vi "Extract the Sine Wave NEW FILTER.vi"() -> ()   [LabVIEW 2019, in "DSP.lvclass"]
doc: "This example demonstrates how a signal can be extracted from bandlimited noise using the filter VIs."
uses:
  DSP.lvclass
  <vilib>/Analysis/3filter.llb/Filter Passband Type.ctl
  <vilib>/Analysis/3filter.llb/IIR Cascade Filter with I.C. (DBL).vi
  <vilib>/Analysis/3filter.llb/IIR Filter with I.C. (DBL).vi
  <vilib>/addons/Digital Filter Design/Process.llb/DFD Filtering with State (Wfm).vi
  <vilib>/addons/Digital Filter Design/Process.llb/DFD Filtering (Wfm NChan).vi
  <vilib>/Analysis/3filter.llb/Butterworth Filter (DBL).vi
  <vilib>/Analysis/NI_AALBase.lvlib
  <vilib>/addons/Digital Filter Design/NI_DigFilterLicensed.lvlib
  <vilib>/measure/NI_MABase.lvlib
panel:
  in  "Q":dbl
  in  "notch (Hz)":dbl
  out "Numeric":i32
  out "Waveform Graph":cluster{dbl, dbl, "Filtered X":dbl[]}[](graph)
  in  "Sample rate (Hz)":dbl=1000.0
  in  "Stop":bool
  in  "Filter Order":i32(slide)=5 scale=0.0..10.0
  in  "Cut-Off Frequency (Hz)":dbl(slide)=20.0 scale=0.0..100.0
  in  "Sine Frequency (Hz)":dbl(slide)=10.0 scale=0.0..200.0
  # "Overview: Removes additive noise from a sinusoid using a lowpass filter.\nRequirements: LabVIEW Full Development System\nInstructions:\n1. Run the VI.\n2. Change the Cut-Off Frequency and Filter Order, noting the effect on the filtered waveform.\n3. Click Stop to stop the VI."
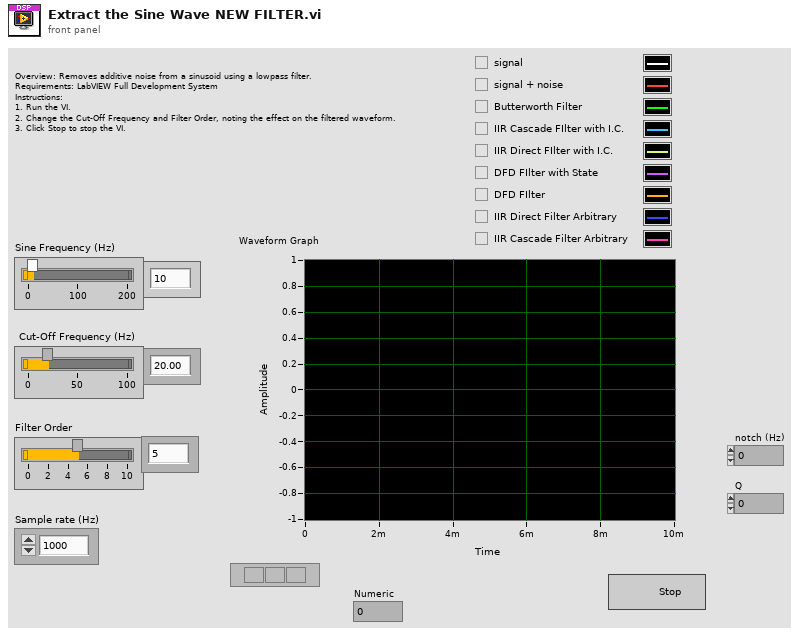
[diagram p1: front panel]
types:
  T1 = cluster{"filter structure":enum32{"IIR 2nd Order", "IIR 4th Order"}, "Reverse Coefficients":dbl[], "Forward Coefficients":dbl[]}
  T2 = enum16{"Sine Wave", "Triangle Wave", "Square Wave", "Sawtooth Wave"}
  T3 = typedef "NI_AALBase.lvlib/Filter Passband Type.ctl" = enum32{"Lowpass", "Highpass", "Bandpass", "Bandstop"}
  T4 = typedef "NI_DigFilterLicensed.lvlib/DFD Filter Obj.ctl" = cluster{"mSRate_Fs":dbl, "mSRate_Version":string, "mSRate_Comments":string, "mSRate_OrgCoef":T5, "mSRate_CurCoef":T5, "mSRate_Quantized?":bool, "mSRate_QCoef":T5, "mSRate_QSettings":T7[], "mSRate_Order":i32, "mSRate_Scaling":cluster{"mSRate_ScaleByPowerOf2?":bool, "mSRate_ScaleType":T9}}
  T5 = typedef "NI_DigFilterLicensed.lvlib/DFD Filter Coef.ctl" = cluster{"type":T6, "gain":dbl, "coef a (k)":dbl[], "coef b (v)":dbl[]}
  T6 = typedef "NI_DigFilterLicensed.lvlib/DFD Filter Structure Type Selector.ctl" = enum16{"Undefined", "FIR Direct Form", "FIR Direct Form Transposed", "FIR Symmetric", "FIR Antisymmetric", "IIR Direct Form I", "IIR Direct Form I Transposed", "IIR Direct Form II", "IIR Direct Form II Transposed", "IIR Cascaded Second Order Sections Form I", "IIR Cascaded Second Order Sections Form I Transposed", "IIR Cascaded Second Order Sections Form II", "IIR Cascaded Second Order Sections Form II Transposed", "Lattice Allpass (basic sections)", "Lattice Allpass (one multiplier sections)", "Lattice Allpass (normalized sections)", "Lattice AR (basic sections)", "Lattice AR (one multiplier sections)", "Lattice AR (normalized sections)", "Lattice MA (minimum phase)", "Lattice MA (maximum phase)", "Lattice ARMA (basic sections)", "Lattice ARMA (one multiplier sections)", "Lattice ARMA (normalized sections)"}
  T7 = typedef "NI_DigFilterLicensed.lvlib/dfd_Internal Quantization Settings.ctl" = cluster{"source":T8, "wl":i16, "iwl":i16, "overflow mode":enum16{"Saturation", "Wrap"}, "rounding mode":enum16{"Nearest", "Truncation"}, "signed?":bool}
  T8 = typedef "NI_DigFilterLicensed.lvlib/dfd_Internal Quantization Srcs.ctl" = u16
  T9 = typedef "NI_DigFilterLicensed.lvlib/DFD Coef Norm Type.ctl" = enum16{"No Norm", "Time Domain 1-Norm", "Time Domain 2-Norm", "Time Domain Inf-Norm"}
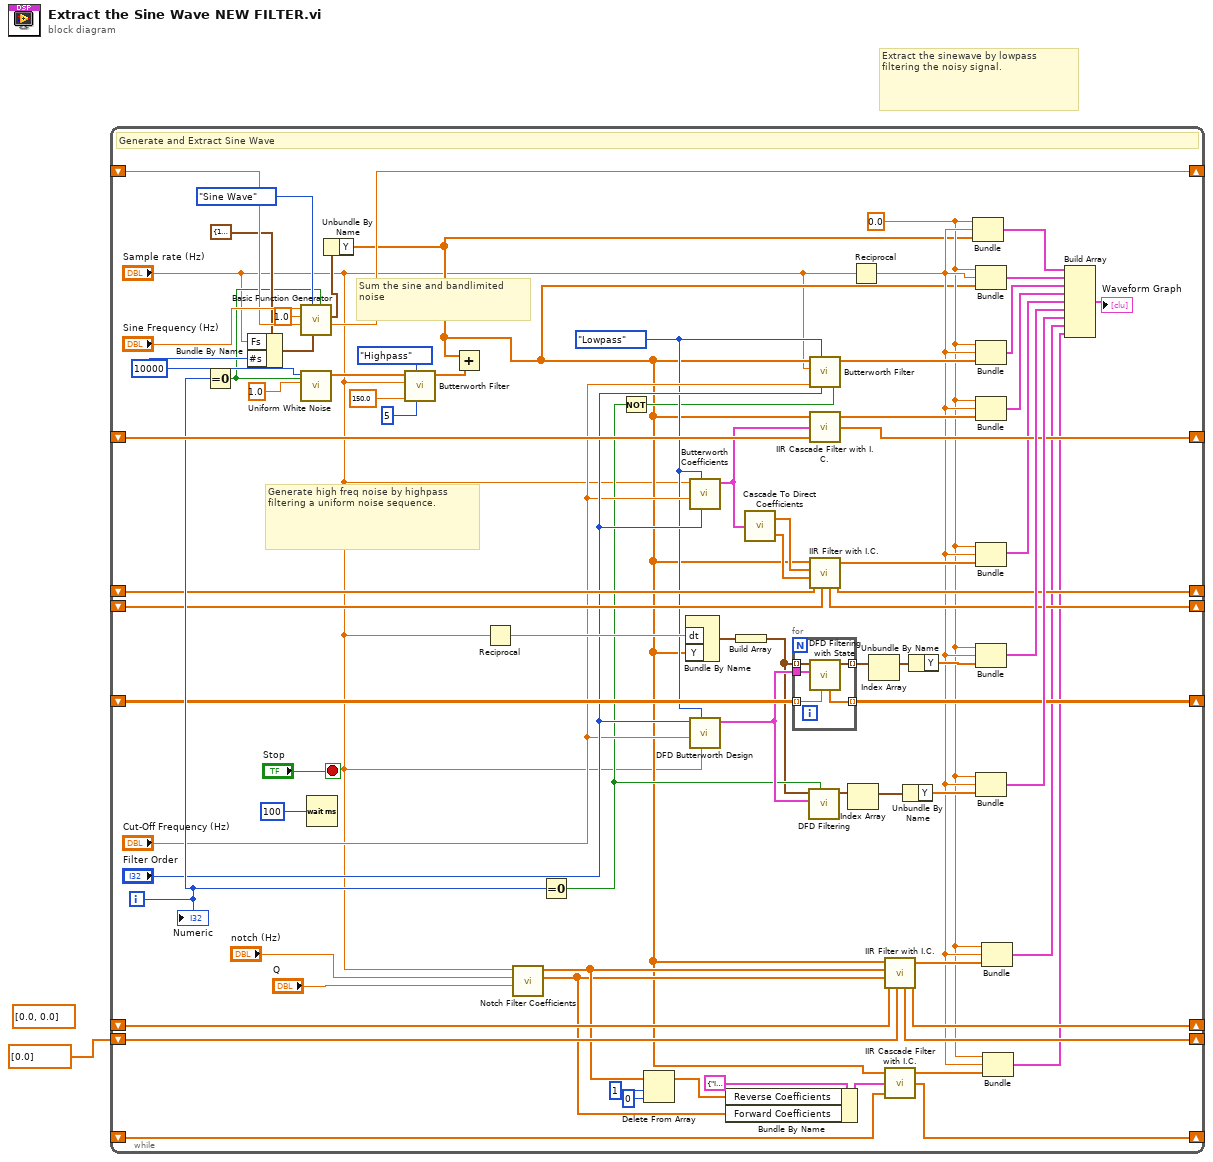
[diagram p0: block diagram]
diagram:
  (unwired) dbl[] [0.0, 0.0] ("Final X Conditions")
  # "Extract the sinewave by lowpass filtering the noisy signal."
  n1 = while {
    shift-right: [w62] -> _
    shift-left: _ -> [w72]
    shift-right: [w64] -> _
    shift-left: _ -> [w63]
    shift-right: [w57] -> _
    shift-left: _ -> [w55]
    shift-right: [w56] -> _
    shift-left: _ -> [w54]
    shift-right: [w23] -> _
    shift-left: _ -> [w35]
    shift-right: [w36] -> _
    shift-left: dbl[] [0.0] ("Final X Conditions") -> [w34]
    shift-right: [w32] -> _
    shift-left: _ -> [w31]
    shift-right: [w5] -> _
    shift-left: _ -> [w17]
    i -> [w71]
    stop <- "Stop" stop-if-true
    w13 = 0.0
    w41 = Filter_Passband_Type."Lowpass" ("filter type")
    w28 = 10000
    # "Sum the sine and bandlimited noise"
    # "Generate high freq noise by highpass filtering a uniform noise sequence."
    # "Generate and Extract Sine Wave"
    n2 = Equal To 0?(x=w71) -> (x = 0?=w24:bool)
    n3 = Bundle By Name(cluster=cluster{"Fs":dbl, "#s":dbl} {"Fs"=1000.0, "#s"=1000.0} ("sampling info"), "Fs"="Sample rate (Hz)", "#s"=w28) -> (w27:cluster{"Fs":dbl, "#s":dbl})
    n4 = call <vilib>:"Basic Function Generator.vi"("reset signal"=w24, "sampling info"=w27, "signal type"=T2."Sine Wave", "phase"=w31, "amplitude"=1.0, "frequency"="Sine Frequency (Hz)") -> ("phase out"=w32:dbl, "signal out"=w25:waveform(dbl))  [unwired: 3 in, 1 out]
    n5 = call <vilib>:"Uniform White Noise.vi"("initialize?"=w24, "amplitude"=1.0, "samples"=w28) -> ("uniform white noise"=w50:dbl[])  [unwired: 7 in, 1 out]
    n6 = Wait (ms)(milliseconds to wait=u32 100) -> ()  [unwired: 1 out]
    n7 = Unbundle By Name(w25) -> ("Y"=w4:dbl[])
    n8 = call-poly <vilib>:"Butterworth Filter.vi"("order"=5, "filter type"=Filter_Passband_Type."Highpass", "low cutoff freq: fl"=150.0, "sampling freq: fs"="Sample rate (Hz)", "X"=w50) -> ("Filtered X"=w49:dbl[])  [unwired: 3 in, 1 out]
    n9 = Add(x=w4, y=w49) -> ()  [unwired: 1 out]
    n10 = Reciprocal(x="Sample rate (Hz)") -> (1/x=w53:dbl)
    n11 = call "Notch Filter Coefficients.vi"("Q"="Q", "notch (Hz)"="notch (Hz)", "Sample rate (Hz)"="Sample rate (Hz)") -> ("Forward Coefficients"=w8:dbl[], "Reverse Coefficients"=w9:dbl[])  [unwired: 7 in]
    n12 = Equal To 0?(x=w71) -> (x = 0?=w39:bool)
    n13 = Not(x=w39) -> (.not. x?=w40:bool)
    n14 = Delete From Array(array=w9, length=1, index=0) -> (array with subset deleted=w12:dbl[])  [unwired: 1 out]
    n15 = Bundle By Name("dt"=w53, "Y"=w4) -> (w7:waveform(dbl))  [unwired: 1 in]
    n16 = call <vilib>:"Butterworth Coefficients.vi"("order"="Filter Order", "filter type"=w41, "low cutoff freq: fl"="Cut-Off Frequency (Hz)", "sampling freq: fs"="Sample rate (Hz)") -> ("IIR Filter Cluster"=w22:T1)  [unwired: 6 in, 1 out]
    n17 = call <vilib>:"DFD Butterworth Design.vi"("fs [Hz]"="Sample rate (Hz)", "filter type"=w41, "low cutoff freq [Hz]"="Cut-Off Frequency (Hz)", "order"="Filter Order") -> ("filter out"=w52:T4)  [unwired: 6 in, 1 out]
    n18 = Bundle By Name(cluster=T1 {"filter structure"=enum."IIR 2nd Order", "Reverse Coefficients"=[], "Forward Coefficients"=[]} ("IIR Filter Cluster"), "Reverse Coefficients"=w12, "Forward Coefficients"=w8) -> (w21:T1)
    n19 = Build Array(w7) -> (w6:waveform(dbl)[])
    n20 = call <vilib>:"Cascade To Direct Coefficients.vi"("IIR Filter Cluster"=w22) -> ("Reverse Coefficients"=w59:dbl[], "Forward Coefficients"=w58:dbl[])
    n21 = for {
      tunnel: [w85] -> w64 mode=indexing
      tunnel: w63 -> [w84] mode=indexing
      tunnel: w52 -> [w83]
      tunnel: w6 -> [w82] mode=indexing
      tunnel: [w81] -> w44 mode=indexing
      n22 = call-poly <vilib>:"DFD Filtering with State.vi"("state in"=w84, "filter"=w83, "signal in"=w82) -> ("signal out"=w81:waveform(dbl), "state out"=w85:dbl[])  [unwired: 6 in, 1 out]
    }
    n23 = call-poly <vilib>:"DFD Filtering.vi"("init? (F)"=w39, "filter"=w52, "signal in"=w6) -> ("signal out"=w46:waveform(dbl)[])  [unwired: 7 in, 1 out]
    n24 = call-poly <vilib>:"Butterworth Filter.vi"("init/cont (init:F)"=w40, "order"="Filter Order", "filter type"=w41, "low cutoff freq: fl"="Cut-Off Frequency (Hz)", "sampling freq: fs"="Sample rate (Hz)", "X"=w4) -> ("Filtered X"=w69:dbl[])  [unwired: 2 in, 1 out]
    n25 = call-poly <vilib>:"IIR Cascade Filter with I.C..vi"("Initial Filter State"=w72, "IIR Filter Cluster"=w22, "X"=w4) -> ("Final Filter State"=w62:dbl[], "Filtered X"=w70:dbl[])  [unwired: 1 out]
    n26 = call-poly <vilib>:"IIR Filter with I.C..vi"("Initial Y Conditions"=w54, "Initial X Conditions"=w55, "Forward Coefficients"=w58, "Reverse Coefficients"=w59, "X"=w4) -> ("Final X Conditions"=w57:dbl[], "Final Y Conditions"=w56:dbl[], "Filtered X"=w60:dbl[])  [unwired: 2 in, 1 out]
    n27 = Index Array(array=w46) -> (element=w48:waveform(dbl))  [unwired: 1 in]
    n28 = Reciprocal(x="Sample rate (Hz)") -> (1/x=w14:dbl)
    n29 = Index Array(array=w44) -> (element=w2:waveform(dbl))  [unwired: 1 in]
    n30 = call-poly <vilib>:"IIR Filter with I.C..vi"("Initial Y Conditions"=w34, "Initial X Conditions"=w35, "Forward Coefficients"=w8, "Reverse Coefficients"=w9, "X"=w4) -> ("Final X Conditions"=w23:dbl[], "Final Y Conditions"=w36:dbl[], "Filtered X"=w38:dbl[])  [unwired: 2 in, 1 out]
    n31 = call-poly <vilib>:"IIR Cascade Filter with I.C..vi"("Initial Filter State"=w17, "IIR Filter Cluster"=w21, "X"=w4) -> ("Final Filter State"=w5:dbl[], "Filtered X"=w15:dbl[])  [unwired: 1 out]
    n32 = Unbundle By Name(w48) -> ("Y"=w47:dbl[])
    n33 = Unbundle By Name(w2) -> ("Y"=w45:dbl[])
    n34 = Bundle(w13, w14, "Y"=w4) -> (w43:cluster{dbl, dbl, "Y":dbl[]})  [unwired: 1 in]
    n35 = Bundle(w13, w14, "Y"=w4) -> (w68:cluster{dbl, dbl, "Y":dbl[]})  [unwired: 1 in]
    n36 = Bundle(w13, w14, "Filtered X"=w69) -> (w79:cluster{dbl, dbl, "Filtered X":dbl[]})  [unwired: 1 in]
    n37 = Bundle(w13, w14, "Filtered X"=w70) -> (w67:cluster{dbl, dbl, "Filtered X":dbl[]})  [unwired: 1 in]
    n38 = Bundle(w13, w14, "Filtered X"=w60) -> (w61:cluster{dbl, dbl, "Filtered X":dbl[]})  [unwired: 1 in]
    n39 = Bundle(w13, w14, "Y"=w45) -> (w66:cluster{dbl, dbl, "Y":dbl[]})  [unwired: 1 in]
    n40 = Bundle(w13, w14, "Y"=w47) -> (w65:cluster{dbl, dbl, "Y":dbl[]})  [unwired: 1 in]
    n41 = Bundle(w13, w14, "Filtered X"=w38) -> (w37:cluster{dbl, dbl, "Filtered X":dbl[]})  [unwired: 1 in]
    n42 = Bundle(w13, w14, "Filtered X"=w15) -> (w16:cluster{dbl, dbl, "Filtered X":dbl[]})  [unwired: 1 in]
    n43 = Build Array(w43, w68, w79, w67, w61, w66, w65, w37, w16) -> (→"Waveform Graph":cluster{dbl, dbl, "Y":dbl[]}[])
    "Numeric" <- w71
  }
